vi "PCO_GetMetaDataExtern.vi"(8 "error in (no error)":errorcluster {"code" format="%x"}, 10 "pBuf":u16[][](array[numeric])=array1x4097[4097 elements], 11 "ph":u64) -> (0 "error out":errorcluster {"code" format="%x"}, 1 "MetaData":T1, 2 "ErrorMessage":i32 format="%x", 3 "ph out":u64)   [LabVIEW 2019, in "SDK.lvlib" / "RecordingControl.lvlib"]
doc: "<b>Description:</b>\nGets the image buffer attached meta data, if available\n\n<b>Supported camera type:</b>\nAll cameras\n\n<b>Descriptor dependency:</b>\nNone"
uses:
  RecordingControl.lvlib
  Structures/Structures.lvlib
  <vilib>/Utility/miscctls.llb/LVDateTimeRec.ctl
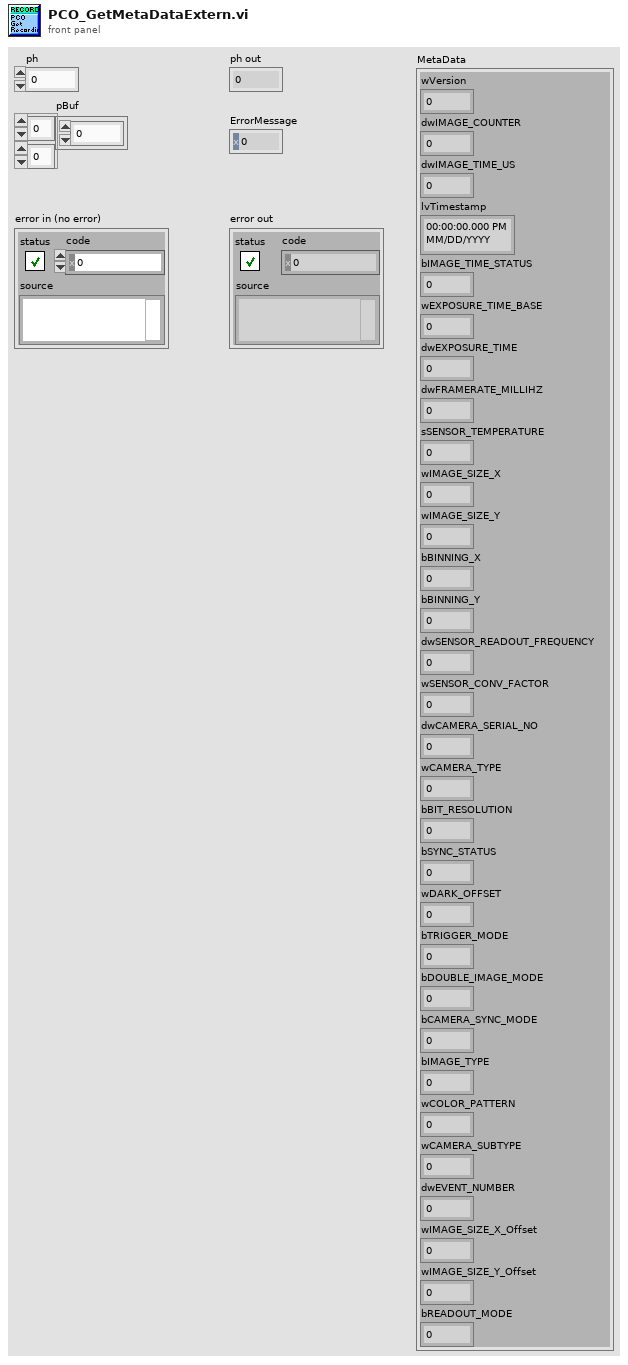
[diagram p1: front panel]
types:
  T1 = cluster{"wVersion":u16, "dwIMAGE_COUNTER":u32, "dwIMAGE_TIME_US":u32, "lvTimestamp":timestamp, "bIMAGE_TIME_STATUS":u8, "wEXPOSURE_TIME_BASE":u16, "dwEXPOSURE_TIME":u32, "dwFRAMERATE_MILLIHZ":u32, "sSENSOR_TEMPERATURE":i16, "wIMAGE_SIZE_X":u16, "wIMAGE_SIZE_Y":u16, "bBINNING_X":u8, "bBINNING_Y":u8, "dwSENSOR_READOUT_FREQUENCY":u32, "wSENSOR_CONV_FACTOR":u16, "dwCAMERA_SERIAL_NO":u32, "wCAMERA_TYPE":u16, "bBIT_RESOLUTION":u8, "bSYNC_STATUS":u8, "wDARK_OFFSET":u16, "bTRIGGER_MODE":u8, "bDOUBLE_IMAGE_MODE":u8, "bCAMERA_SYNC_MODE":u8, "bIMAGE_TYPE":u8, "wCOLOR_PATTERN":u16, "wCAMERA_SUBTYPE":u16, "dwEVENT_NUMBER":u32, "wIMAGE_SIZE_X_Offset":u16, "wIMAGE_SIZE_Y_Offset":u16, "bREADOUT_MODE":u8}
  T2 = typedef "LVDateTimeRec.ctl" = cluster{"fractional second":dbl, "second":i32, "minute":i32, "hour":i32, "day of month":i32, "month":i32, "year":i32, "day of week":i32, "day of year":i32, "DST":i32}
  T3 = cluster{"wSize":u16, "wVersion":u16, "bIMAGE_COUNTER_BCD":cluster{u8, u8, u8, u8}, "bIMAGE_TIME_US_BCD":cluster{u8, u8, u8}, "bIMAGE_TIME_SEC_BCD":u8, "bIMAGE_TIME_MIN_BCD":u8, "bIMAGE_TIME_HOUR_BCD":u8, "bIMAGE_TIME_DAY_BCD":u8, "bIMAGE_TIME_MON_BCD":u8, "bIMAGE_TIME_YEAR_BCD":u8, "bIMAGE_TIME_STATUS":u8, "wEXPOSURE_TIME_BASE":u16, "dwEXPOSURE_TIME":u32, "dwFRAMERATE_MILLIHZ":u32, "sSENSOR_TEMPERATURE":i16, "wIMAGE_SIZE_X":u16, "wIMAGE_SIZE_Y":u16, "bBINNING_X":u8, "bBINNING_Y":u8, "dwSENSOR_READOUT_FREQUENCY":u32, "wSENSOR_CONV_FACTOR":u16, "dwCAMERA_SERIAL_NO":u32, "wCAMERA_TYPE":u16, "bBIT_RESOLUTION":u8, "bSYNC_STATUS":u8, "wDARK_OFFSET":u16, "bTRIGGER_MODE":u8, "bDOUBLE_IMAGE_MODE":u8, "bCAMERA_SYNC_MODE":u8, "bIMAGE_TYPE":u8, "wCOLOR_PATTERN":u16, "wCAMERA_SUBTYPE":u16, "dwEVENT_NUMBER":u32, "wIMAGE_SIZE_X_Offset":u16, "wIMAGE_SIZE_Y_Offset":u16, "bREADOUT_MODE":u8}
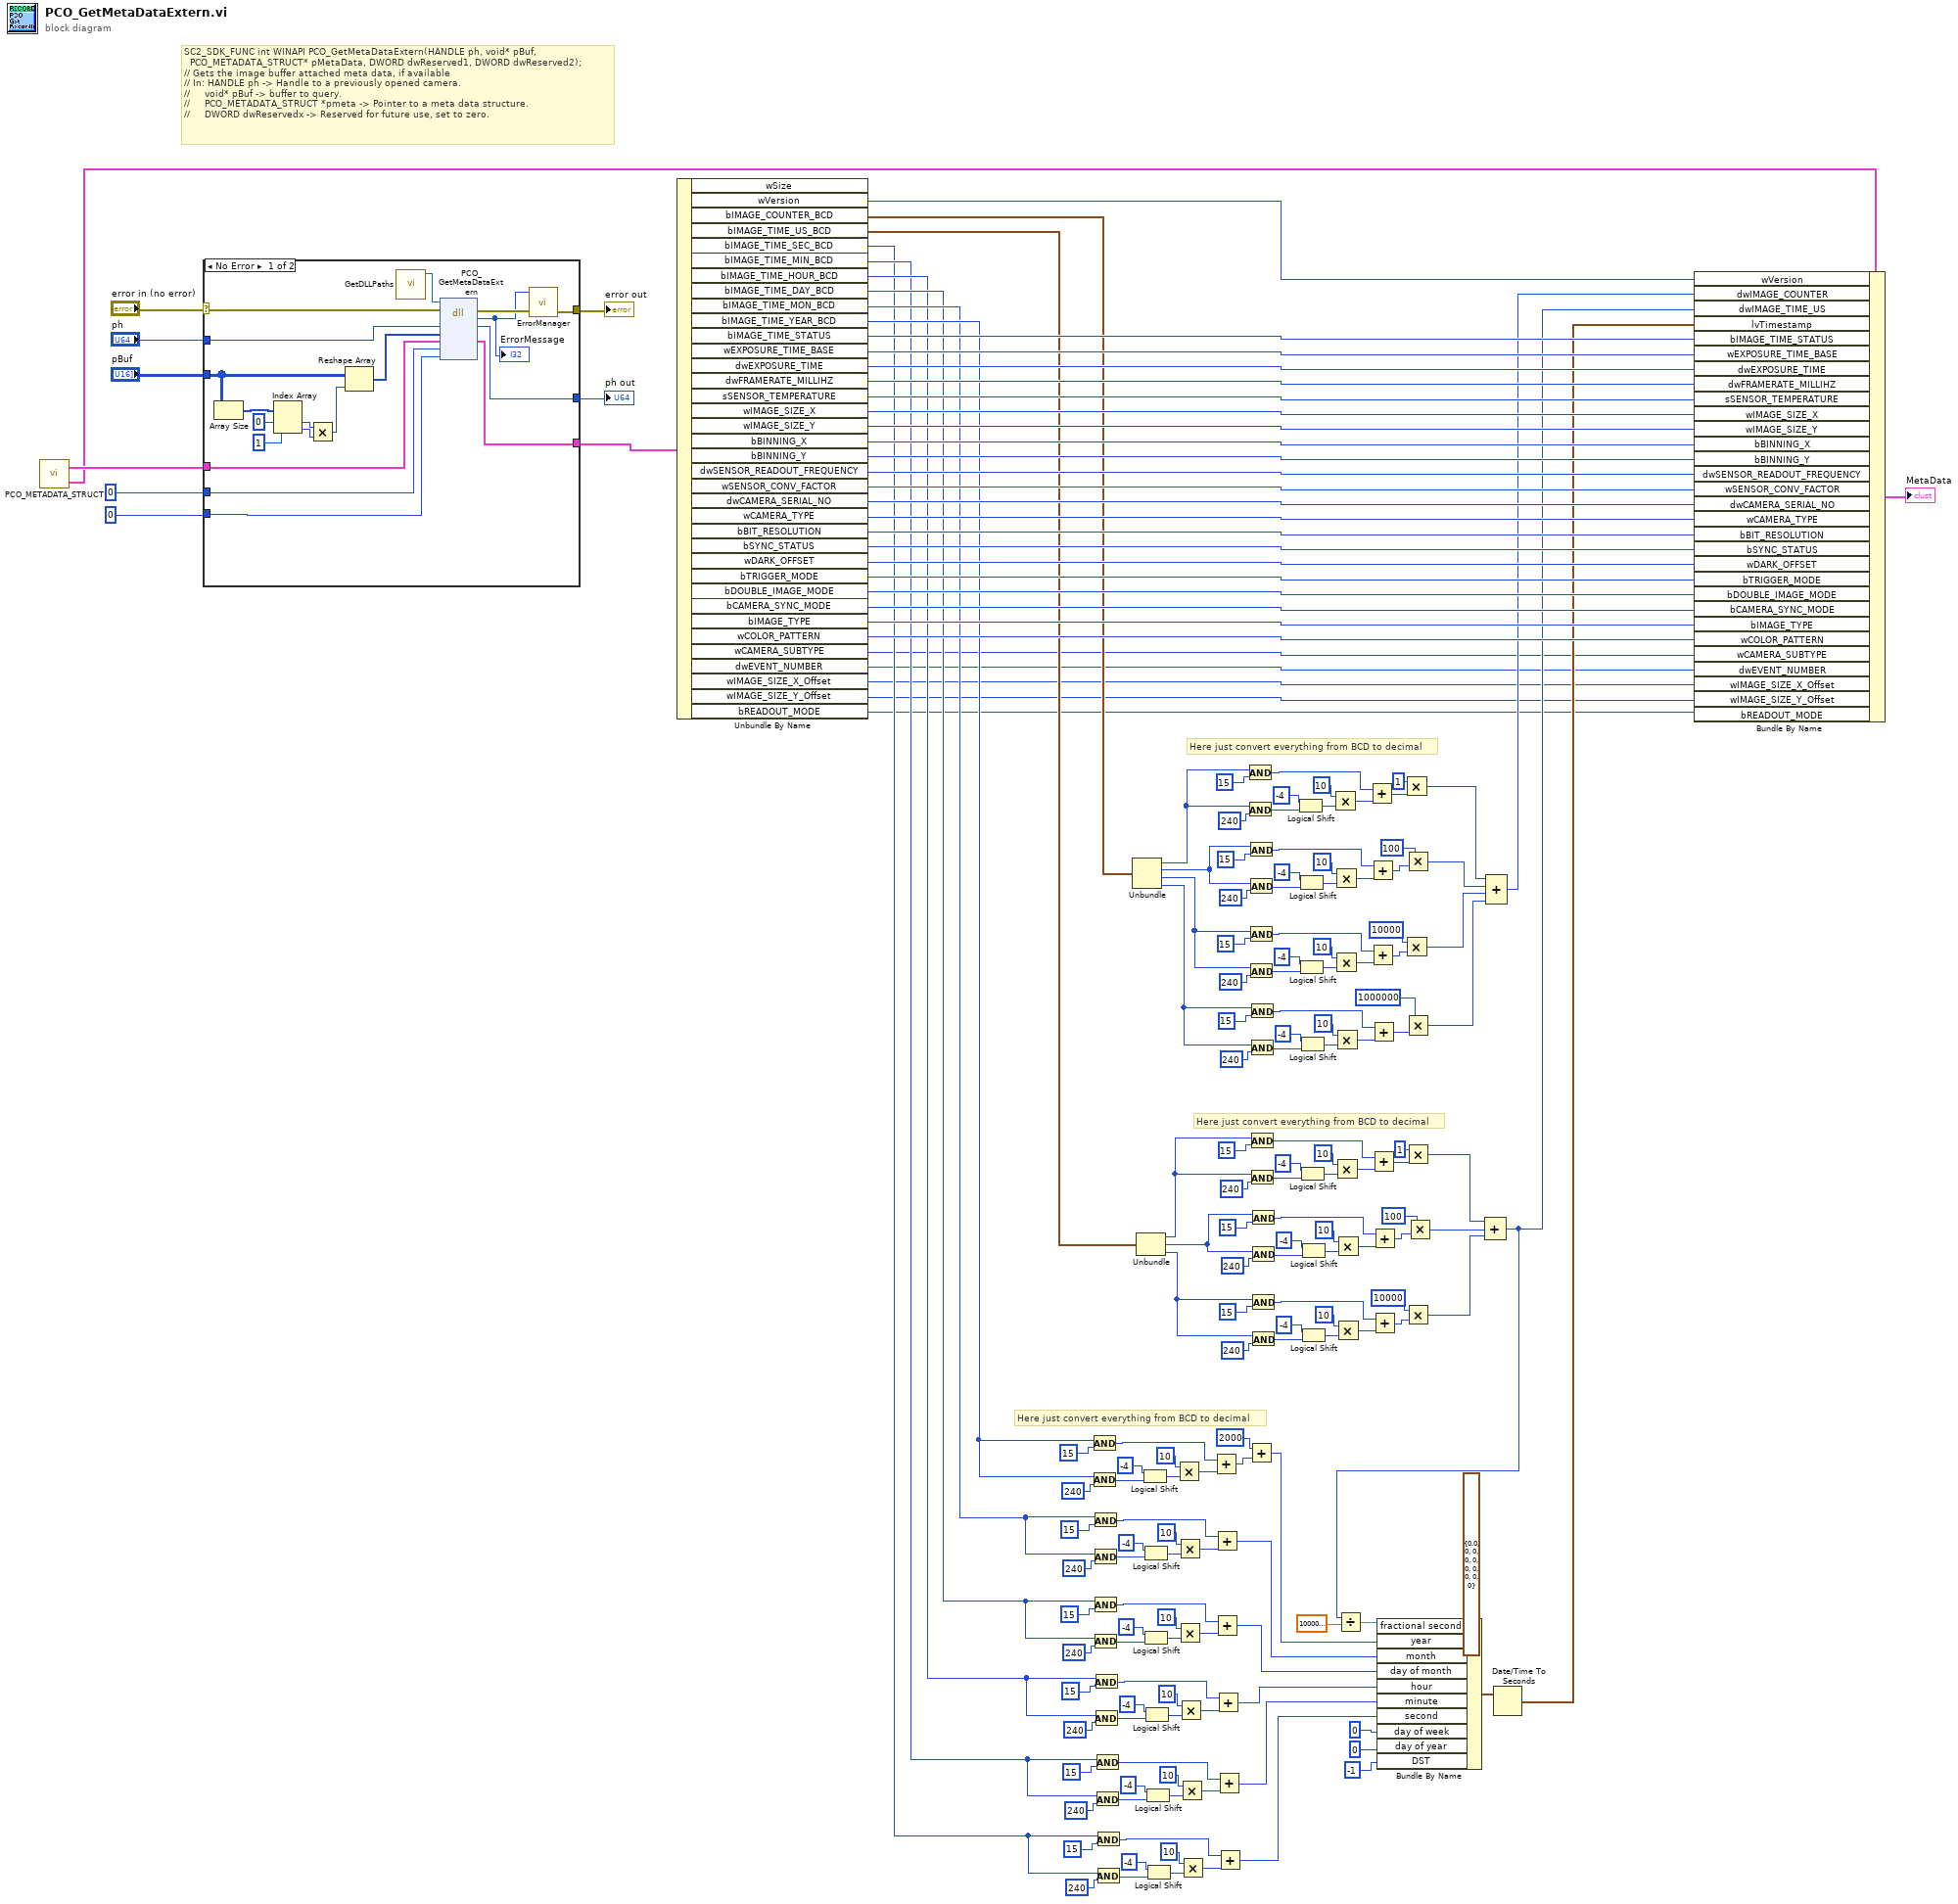
[diagram p0: block diagram]
diagram:
  # "Here just convert everything from BCD to decimal"
  # "Here just convert everything from BCD to decimal"
  # "Here just convert everything from BCD to decimal"
  # "SC2_SDK_FUNC int WINAPI PCO_GetMetaDataExtern(HANDLE ph, void* pBuf,\n  PCO_METADATA_STRUCT* pMetaData, DWORD dwReserved1, DWORD dwReserved2);\n// Gets the image buffer attached meta data, if available\n// In: HANDLE ph -> Handle to a previously opened camera.\n//     void* pBuf -> buffer to query.\n//     PCO_METADATA_STRUCT *pmeta -> Pointer to a meta data structure.\n//     DWORD dwReservedx -> Reserved for future use, set to zero."
  n1 = call "PCO_METADATA_STRUCT.vi"() -> ("PCO_METADATA_STRUCT"=w9:T1, "PCO_METADATA_STRUCT_Raw"=w192:T3)  [unwired: 4 in, 2 out]
  n2 = case shown="No Error" "error in (no error)" {
    selector: "error in (no error)" -> [w211 w218]
    tunnel: "ph" -> [w215 w217]
    tunnel: [w214 w217] -> w195
    tunnel: w192 -> [w213 w216]
    tunnel: [w212 w216] -> w8
    tunnel: [w209 w218] -> w194
    tunnel: u32 0 ("dwReserved1") -> [w206 _]
    tunnel: u32 0 ("dwReserved1") -> [w205 _]
    tunnel: "pBuf" -> [w199 _]
    frame No Error {
      n3 = Array Size(array=w199) -> (size(s)=w200:i32[])
      n4 = Index Array(array=w200, index #1=0 ("index"), index #2=1 ("index")) -> (element #1=w203:i32, element #2=w204:i32)
      n5 = Multiply(x=w203, y=w204) -> (x*y=w198:i32)
      n6 = Reshape Array(w199, w198) -> (w197:u16[])
      n7 = call "GetDLLPaths.vi"() -> ("SC2_Cam_Path"=w207:path)  [unwired: 8 in, 3 out]
      n8 = dll-call lib="?" fn="PCO_GetMetaDataExtern"(path in=w207, error in=w211, "ph"=w215, "pBuf"=w197, "pMetaData"=w213, "dwReserved1"=w206, "dwReserved2"=w205) -> (error out=w210:errorcluster, "return type"=w208:i32, "ph"=w214:u64, "pMetaData"=w212:T3)  [unwired: 4 in, 1 out]
      "ErrorMessage" <- w208
      n9 = call "ErrorManager.vi"("error in (no error)"=w210, "error code"=w208) -> ("error out"=w209:errorcluster)  [unwired: 2 in, 1 out]
    }
    frame Error {
    }
  }
  "ph out" <- w195
  "error out" <- w194
  n10 = Unbundle By Name(w8) -> ("wVersion"=w189:u16, "bIMAGE_COUNTER_BCD"=w102:cluster{u8, u8, u8, u8}, "bIMAGE_TIME_US_BCD"=w24:cluster{u8, u8, u8}, "bIMAGE_TIME_SEC_BCD"=w114:u8, "bIMAGE_TIME_MIN_BCD"=w115:u8, "bIMAGE_TIME_HOUR_BCD"=w116:u8, "bIMAGE_TIME_DAY_BCD"=w117:u8, "bIMAGE_TIME_MON_BCD"=w118:u8, "bIMAGE_TIME_YEAR_BCD"=w163:u8, "bIMAGE_TIME_STATUS"=w185:u8, "wEXPOSURE_TIME_BASE"=w184:u16, "dwEXPOSURE_TIME"=w183:u32, "dwFRAMERATE_MILLIHZ"=w182:u32, "sSENSOR_TEMPERATURE"=w181:i16, "wIMAGE_SIZE_X"=w180:u16, "wIMAGE_SIZE_Y"=w179:u16, "bBINNING_X"=w178:u8, "bBINNING_Y"=w177:u8, "dwSENSOR_READOUT_FREQUENCY"=w176:u32, "wSENSOR_CONV_FACTOR"=w175:u16, "dwCAMERA_SERIAL_NO"=w174:u32, "wCAMERA_TYPE"=w173:u16, "bBIT_RESOLUTION"=w172:u8, "bSYNC_STATUS"=w171:u8, "wDARK_OFFSET"=w170:u16, "bTRIGGER_MODE"=w169:u8, "bDOUBLE_IMAGE_MODE"=w168:u8, "bCAMERA_SYNC_MODE"=w167:u8, "bIMAGE_TYPE"=w166:u8, "wCOLOR_PATTERN"=w165:u16, "wCAMERA_SUBTYPE"=w6:u16, "dwEVENT_NUMBER"=w5:u32, "wIMAGE_SIZE_X_Offset"=w4:u16, "wIMAGE_SIZE_Y_Offset"=w3:u16, "bREADOUT_MODE"=w2:u8)  [unwired: 1 out]
  n11 = And(x=w163, y=u8 15) -> (x .and. y?=w159:u8)
  n12 = And(x=w163, y=u8 240) -> (x .and. y?=w186:u8)
  n13 = And(x=w118, y=u8 15) -> (x .and. y?=w158:u8)
  n14 = And(x=w118, y=u8 240) -> (x .and. y?=w153:u8)
  n15 = And(x=w117, y=u8 15) -> (x .and. y?=w142:u8)
  n16 = And(x=w117, y=u8 240) -> (x .and. y?=w137:u8)
  n17 = And(x=w116, y=u8 15) -> (x .and. y?=w143:u8)
  n18 = And(x=w116, y=u8 240) -> (x .and. y?=w148:u8)
  n19 = And(x=w115, y=u8 15) -> (x .and. y?=w127:u8)
  n20 = And(x=w115, y=u8 240) -> (x .and. y?=w132:u8)
  n21 = And(x=w114, y=u8 15) -> (x .and. y?=w126:u8)
  n22 = And(x=w114, y=u8 240) -> (x .and. y?=w121:u8)
  n23 = Unbundle(w102) -> (w32:u8, w31:u8, w30:u8, w29:u8)
  n24 = Unbundle(w24) -> (w23:u8, w22:u8, w21:u8)
  n25 = Logical Shift(y=i16 -4, x=w186) -> (x << y=w162:u8)
  n26 = Logical Shift(y=i16 -4, x=w153) -> (x << y=w155:u8)
  n27 = Logical Shift(y=i16 -4, x=w137) -> (x << y=w139:u8)
  n28 = Logical Shift(y=i16 -4, x=w148) -> (x << y=w146:u8)
  n29 = Logical Shift(y=i16 -4, x=w132) -> (x << y=w130:u8)
  n30 = Logical Shift(y=i16 -4, x=w121) -> (x << y=w123:u8)
  n31 = Multiply(x=u8 10, y=w162) -> (x*y=w160:u8)
  n32 = Multiply(x=u8 10, y=w155) -> (x*y=w157:u8)
  n33 = Multiply(x=u8 10, y=w139) -> (x*y=w141:u8)
  n34 = Multiply(x=u8 10, y=w146) -> (x*y=w144:u8)
  n35 = Multiply(x=u8 10, y=w130) -> (x*y=w128:u8)
  n36 = Multiply(x=u8 10, y=w123) -> (x*y=w125:u8)
  n37 = Add(x=w159, y=w160) -> (x+y=w15:u8)
  n38 = Add(x=w158, y=w157) -> (x+y=w108:u8)
  n39 = Add(x=w142, y=w141) -> (x+y=w107:u8)
  n40 = Add(x=w143, y=w144) -> (x+y=w106:u8)
  n41 = Add(x=w127, y=w128) -> (x+y=w105:u8)
  n42 = Add(x=w126, y=w125) -> (x+y=w104:u8)
  n43 = And(x=w32, y=u8 15) -> (x .and. y?=w77:u8)
  n44 = And(x=w32, y=u8 240) -> (x .and. y?=w72:u8)
  n45 = And(x=w31, y=u8 15) -> (x .and. y?=w78:u8)
  n46 = And(x=w31, y=u8 240) -> (x .and. y?=w83:u8)
  n47 = And(x=w30, y=u8 15) -> (x .and. y?=w94:u8)
  n48 = And(x=w30, y=u8 240) -> (x .and. y?=w99:u8)
  n49 = Add(x=2000, y=w15) -> (x+y=w13:i32)
  n50 = And(x=w29, y=u8 15) -> (x .and. y?=w93:u8)
  n51 = And(x=w29, y=u8 240) -> (x .and. y?=w88:u8)
  n52 = And(x=w23, y=u8 15) -> (x .and. y?=w48:u8)
  n53 = And(x=w23, y=u8 240) -> (x .and. y?=w53:u8)
  n54 = And(x=w22, y=u8 15) -> (x .and. y?=w47:u8)
  n55 = And(x=w22, y=u8 240) -> (x .and. y?=w42:u8)
  n56 = And(x=w21, y=u8 15) -> (x .and. y?=w39:u8)
  n57 = And(x=w21, y=u8 240) -> (x .and. y?=w34:u8)
  n58 = Logical Shift(y=i16 -4, x=w72) -> (x << y=w74:u8)
  n59 = Logical Shift(y=i16 -4, x=w83) -> (x << y=w81:u8)
  n60 = Logical Shift(y=i16 -4, x=w99) -> (x << y=w97:u8)
  n61 = Logical Shift(y=i16 -4, x=w88) -> (x << y=w90:u8)
  n62 = Logical Shift(y=i16 -4, x=w53) -> (x << y=w51:u8)
  n63 = Logical Shift(y=i16 -4, x=w42) -> (x << y=w44:u8)
  n64 = Logical Shift(y=i16 -4, x=w34) -> (x << y=w36:u8)
  n65 = Multiply(x=u8 10, y=w74) -> (x*y=w76:u8)
  n66 = Multiply(x=u8 10, y=w81) -> (x*y=w79:u8)
  n67 = Multiply(x=u8 10, y=w97) -> (x*y=w95:u8)
  n68 = Multiply(x=u8 10, y=w90) -> (x*y=w92:u8)
  n69 = Multiply(x=u8 10, y=w51) -> (x*y=w49:u8)
  n70 = Multiply(x=u8 10, y=w44) -> (x*y=w46:u8)
  n71 = Multiply(x=u8 10, y=w36) -> (x*y=w38:u8)
  n72 = Add(x=w77, y=w76) -> (x+y=w66:u8)
  n73 = Add(x=w78, y=w79) -> (x+y=w69:u8)
  n74 = Add(x=w94, y=w95) -> (x+y=w68:u8)
  n75 = Add(x=w93, y=w92) -> (x+y=w67:u8)
  n76 = Add(x=w48, y=w49) -> (x+y=w58:u8)
  n77 = Add(x=w47, y=w46) -> (x+y=w56:u8)
  n78 = Add(x=w39, y=w38) -> (x+y=w57:u8)
  n79 = Multiply(x=u32 1, y=w66) -> (x*y=w28:u32)
  n80 = Multiply(x=u32 10000, y=w68) -> (x*y=w26:u32)
  n81 = Multiply(x=u32 100, y=w69) -> (x*y=w27:u32)
  n82 = Multiply(x=u32 1000000, y=w67) -> (x*y=w25:u32)
  n83 = Multiply(x=u32 1, y=w58) -> (x*y=w19:u32)
  n84 = Multiply(x=u32 10000, y=w57) -> (x*y=w17:u32)
  n85 = Multiply(x=u32 100, y=w56) -> (x*y=w18:u32)
  n86 = Compound Arithmetic op=ADD(w19, w18, w17) -> (w11:u32)
  n87 = Divide(x=w11, y=1000000.0 ("fractional second")) -> (x/y=w10:dbl)
  n88 = Bundle By Name(cluster=T2 {"fractional second"=0.0, "second"=0, "minute"=0, "hour"=0, "day of month"=0, "month"=0, "year"=0, "day of week"=0, "day of year"=0, "DST"=0} ("date time rec"), "fractional second"=w10, "year"=w13, "month"=w108, "day of month"=w107, "hour"=w106, "minute"=w105, "second"=w104, "day of week"=0, "day of year"=0, "DST"=-1) -> (w109:T2)
  n89 = Compound Arithmetic op=ADD(w28, w27, w26, w25) -> (w16:u32)
  n90 = Date/Time To Seconds(2:w109) -> (0:w103:timestamp)  [unwired: 1 in]
  n91 = Bundle By Name(cluster=w9, "wVersion"=w189, "dwIMAGE_COUNTER"=w16, "dwIMAGE_TIME_US"=w11, "lvTimestamp"=w103, "bIMAGE_TIME_STATUS"=w185, "wEXPOSURE_TIME_BASE"=w184, "dwEXPOSURE_TIME"=w183, "dwFRAMERATE_MILLIHZ"=w182, "sSENSOR_TEMPERATURE"=w181, "wIMAGE_SIZE_X"=w180, "wIMAGE_SIZE_Y"=w179, "bBINNING_X"=w178, "bBINNING_Y"=w177, "dwSENSOR_READOUT_FREQUENCY"=w176, "wSENSOR_CONV_FACTOR"=w175, "dwCAMERA_SERIAL_NO"=w174, "wCAMERA_TYPE"=w173, "bBIT_RESOLUTION"=w172, "bSYNC_STATUS"=w171, "wDARK_OFFSET"=w170, "bTRIGGER_MODE"=w169, "bDOUBLE_IMAGE_MODE"=w168, "bCAMERA_SYNC_MODE"=w167, "bIMAGE_TYPE"=w166, "wCOLOR_PATTERN"=w165, "wCAMERA_SUBTYPE"=w6, "dwEVENT_NUMBER"=w5, "wIMAGE_SIZE_X_Offset"=w4, "wIMAGE_SIZE_Y_Offset"=w3, "bREADOUT_MODE"=w2) -> (→"MetaData":T1)
